vi "Enviro.vi"() -> ()   [LabVIEW 2016]
uses:
  <vilib>/addons/database/NI_Database_API.lvlib
panel:
  in  "stop 2":bool
  out "error out":errorcluster
  in  "stop":bool
  in  "error in (no error)":errorcluster
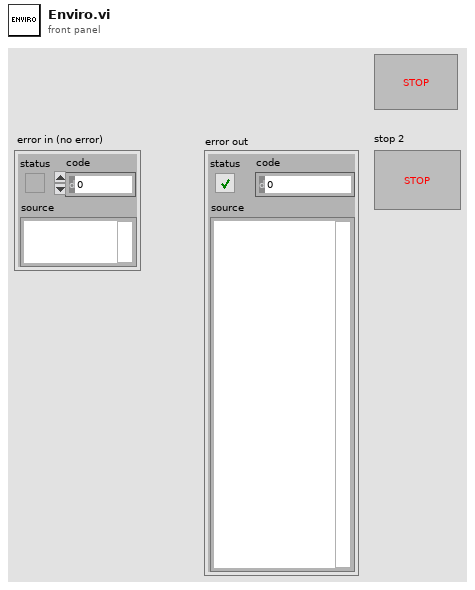
[diagram p1: front panel]
types:
  T1 = typedef "NI_Database_API.lvlib/Conn ObjectReference.ctl" = refnum<k1>
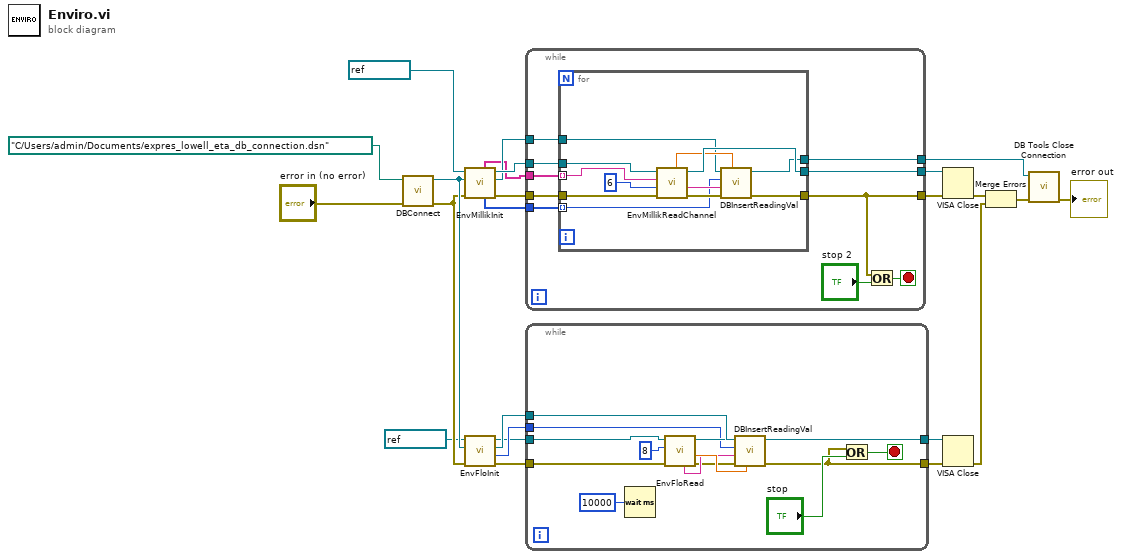
[diagram p0: block diagram]
diagram:
  n1 = call "DBConnect.vi"("error in (no error)"="error in (no error)", "connection path"=path "C:/Users/admin/Documents/expres_lowell_eta_db_connection.dsn" ("connection information")) -> ("error out"=w12:errorcluster, "db connection out"=w13:T1)  [unwired: 8 in]
  n2 = call "EnvMillikInit.vi"("error in (no error)"=w12, "db connection in"=w13, "VISA Refnum in"=refnum<visa-resource-name> "COM6" ("VISA resource name")) -> ("error out"=w19:errorcluster, "db connection out"=w17:T1, "VISA Refnum out"=w18:refnum<visa-resource-name>, "sensor id array out"=w14:i32[], "channel array out"=w16:string[])  [unwired: 4 in]
  n3 = call "EnvFloInit.vi"("error in (no error)"=w12, "db connection in"=w13, "VISA Refnum in"=refnum<visa-resource-name> "COM5") -> ("error out"=w4:errorcluster, "sensor id"=w6:i32, "db connection out"=w7:T1, "VISA Refnum out"=w3:refnum<visa-resource-name>)  [unwired: 5 in]
  n4 = while {
    tunnel: w16 -> [w31]
    tunnel: w18 -> [w32]
    tunnel: [w34] -> w22
    tunnel: w19 -> [w33]
    tunnel: w17 -> [w28]
    tunnel: [w26] -> w15
    tunnel: [w27] -> w11
    tunnel: w14 -> [w25]
    stop <- w30 stop-if-true
    n5 = for {
      tunnel: w31 -> [w37] mode=indexing
      tunnel: w32 -> [w44]
      tunnel: [w46] -> w34
      tunnel: w33 -> [w45]
      tunnel: w28 -> [w42]
      tunnel: [w40] -> w26
      tunnel: [w39] -> w27
      tunnel: w25 -> [w35] mode=indexing
      n6 = call "EnvMillikReadChannel.vi"("error in (no error)"=w45, "timeout"=6, "channel"=w37, "VISA Refnum in"=w44) -> ("error out"=w41:errorcluster, "timestamp"=w38:string, "VISA Refnum out"=w46:refnum<visa-resource-name>, "value"=w43:dbl)  [unwired: 3 in, 1 out]
      n7 = call "DBInsertReadingVal.vi"("db connection in"=w42, "sensor id"=w35, "timestamp"=w38, "error in (no error)"=w41, "reading value"=w43) -> ("db connection out"=w39:T1, "error out"=w40:errorcluster)  [unwired: 4 in]
    }
    n8 = Or(x=w26, y="stop 2") -> (x .or. y?=w30:bool)
  }
  n9 = while {
    tunnel: w6 -> [w48]
    tunnel: w4 -> [w58]
    tunnel: [w49] -> w1
    tunnel: w7 -> [w59]
    tunnel: w3 -> [w57]
    tunnel: [w55] -> w2
    stop <- w50 stop-if-true
    n10 = Wait (ms)(milliseconds to wait=u32 10000) -> ()  [unwired: 1 out]
    n11 = call "EnvFloRead.vi"("error in (no error)"=w58, "read byte count"=u32 8, "VISA Refnum in"=w57) -> ("error out"=w52:errorcluster, "value"=w54:dbl, "VISA Refnum out"=w55:refnum<visa-resource-name>, "timestamp"=w53:string)  [unwired: 3 in, 2 out]
    n12 = call "DBInsertReadingVal.vi"("db connection in"=w59, "sensor id"=w48, "timestamp"=w53, "error in (no error)"=w52, "reading value"=w54) -> ("error out"=w49:errorcluster)  [unwired: 4 in, 1 out]
    n13 = Or(x=w49, y="stop") -> (x .or. y?=w50:bool)
  }
  n14 = VISA Close(VISA resource name=w22, error in (no error)=w15) -> (error out=w10:errorcluster)
  n15 = VISA Close(VISA resource name=w2, error in (no error)=w1) -> (error out=w9:errorcluster)
  n16 = Merge Errors(w10, w9) -> (w8:errorcluster)
  n17 = call <vilib>:"DB Tools Close Connection.vi"("error in (no error)"=w8, "connection reference"=w11) -> ("error out"=→"error out":errorcluster)  [unwired: 5 in]
